vi "Teleop.vi"(10 "Match Info":T1={"Autonomous Elapsed Seconds"=0.0, "TeleOp Elapsed Seconds"=0.0, "Disabled Elapsed Seconds"=0.0, "Visited Autonomous"=FALSE, "Visited TeleOp"=FALSE, "Visited Disabled"=FALSE, "Autonomous Settings"={"Autonomous Style"=enum."Independent", "VI Refnum"=refnum}}, 11 "Call Context":T2) -> ()   [LabVIEW 2020]
doc: "This VI is called for each TeleOp packet received from the DS where the robot is not disabled. It is often used to read from the joysticks and update I/O or to update setpoints for timed control loops. It should complete and return within 20 milliseconds or it may miss DS packets."
uses:
  <vilib>/Rock Robotics/Network Tables/NT Read Boolean.vi
  <vilib>/Rock Robotics/Network Tables/NT Read Number.vi
  Robot Global Data.vi
  <vilib>/Rock Robotics/Network Tables/NT Write Numeric Array.vi
  <vilib>/Rock Robotics/WPI/ThirdParty/Phoenix-LabVIEW/Motor Controller/Controls/CTRE_Phoenix_MotorControl_ControlMode.ctl
  <vilib>/Rock Robotics/WPI/Solenoid/Deprecated/WPI_SolenoidSetBool.vi
  <vilib>/Rock Robotics/WPI/Solenoid/WPI_SolenoidValue.ctl
  <vilib>/Rock Robotics/Network Tables/NT Write Number.vi
  <vilib>/Rock Robotics/Network Tables/NT Write Boolean Array.vi
  <vilib>/Rock Robotics/WPI/Solenoid/WPI_SolenoidSetEnum.vi
  <vilib>/Rock Robotics/WPI/Solenoid/Deprecated/WPI_SolenoidGetBool.vi
  <vilib>/Rock Robotics/WPI/DriverStation/WPI_DriverStationMatch Info.ctl
  <vilib>/Rock Robotics/WPI/DriverStation/WPI_DriverStationDerivedRobotMode.ctl
panel:
  out "TargetValid 5":bool
  out "TargetValid 4":bool
  out "POVs":i16[](array[numeric])
  out "Sample Slider 0":dbl(slide) scale=0.0..5.0
  out "Sample Boolean 1":bool
  out "Sample Boolean 0":bool
  # "April tags"
  # "Retroreflective tape"
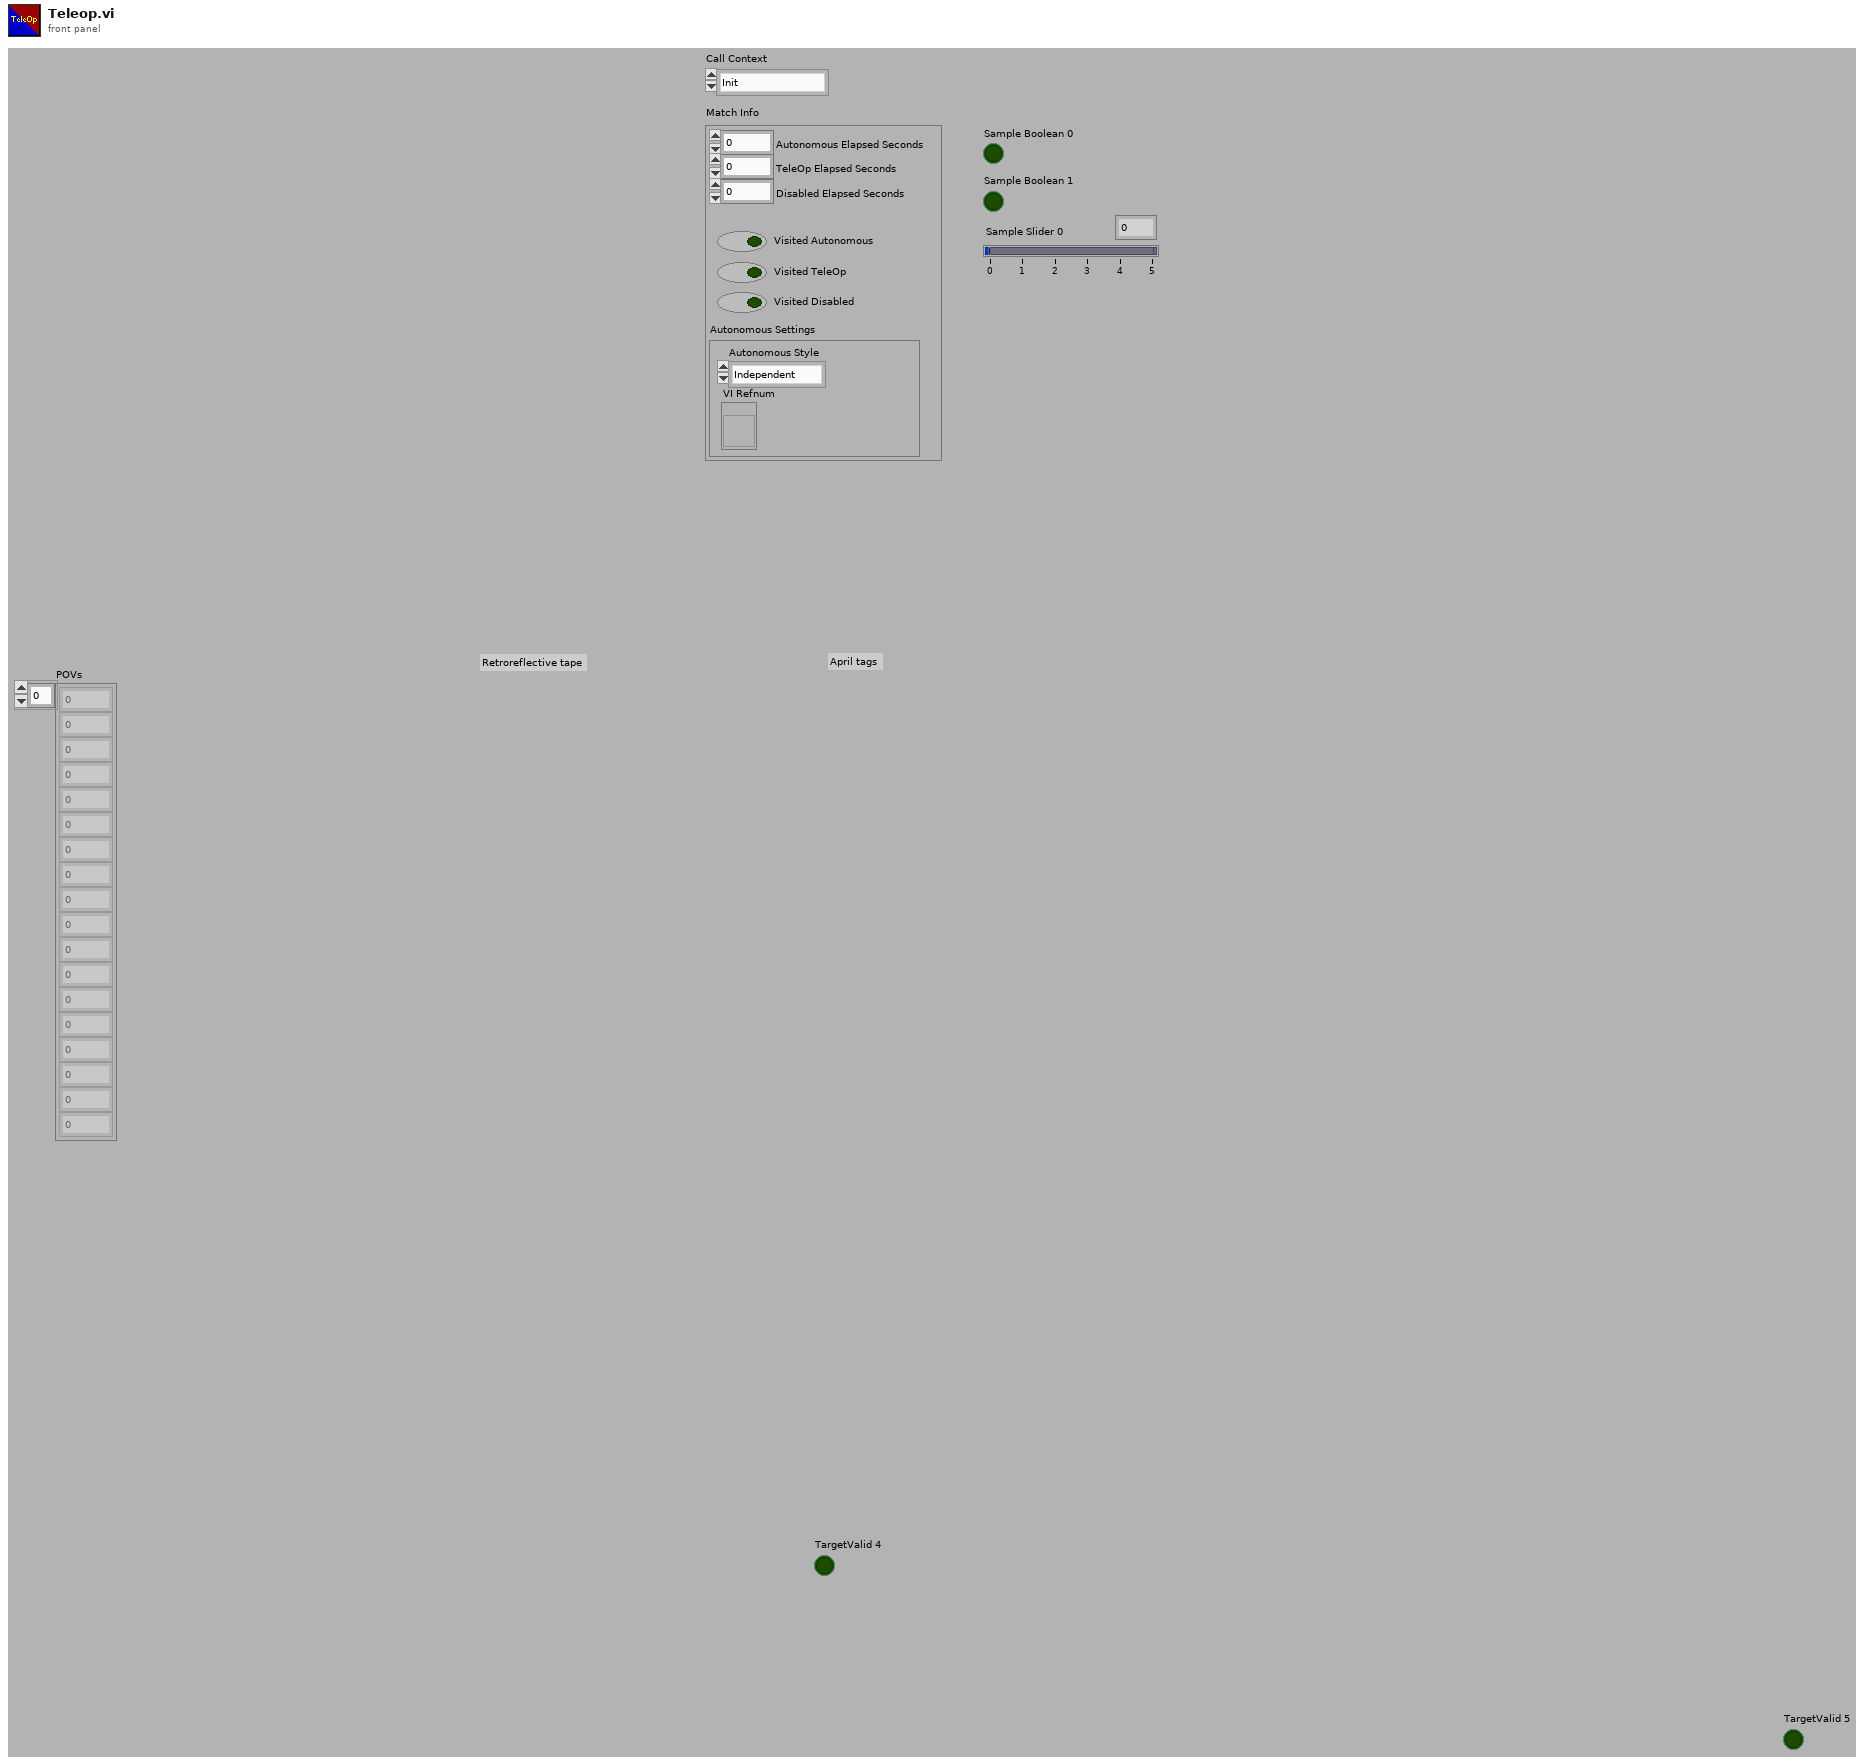
[diagram p1: front panel]
types:
  T1 = typedef "WPI_DriverStationMatch Info.ctl" = cluster{"Autonomous Elapsed Seconds":dbl, "TeleOp Elapsed Seconds":dbl, "Disabled Elapsed Seconds":dbl, "Visited Autonomous":bool, "Visited TeleOp":bool, "Visited Disabled":bool, "Autonomous Settings":cluster{"Autonomous Style":enum16{"Iterative", "Independent"}, "VI Refnum":refnum<vi>}}
  T2 = typedef "WPI_DriverStationDerivedRobotMode.ctl" = enum16{"Init", "Execute", "Stop"}
  T3 = typedef "WPI_SolenoidValue.ctl" = enum16{"Off", "On", "Forward", "Reverse"}
  T4 = cluster{"offsetAngle H":dbl, "offsetAngle V":dbl, "area":dbl, "skew":dbl}
  T5 = typedef "WPI_JoystickDevRef.ctl" = cluster{"Device":T6}
  T6 = typedef "WPI_JoystickDeviceEnum.ctl" = enum16{"USB 0", "USB 1", "USB 2", "USB 3", "USB 4", "USB 5"}
  T7 = cluster{"Buttons[0]":bool, "Buttons[1]":bool, "Buttons[2]":bool, "Buttons[3]":bool, "Buttons[4]":bool, "Buttons[5]":bool, "Buttons[6]":bool, "Buttons[7]":bool, "Buttons[8]":bool}
  T8 = cluster{"Axes[0]":dbl, "Axes[1]":dbl, "Axes[2]":dbl, "Axes[3]":dbl, "Axes[4]":dbl, "Axes[5]":dbl, "Axes[6]":dbl, "Axes[7]":dbl, "Axes[8]":dbl}
  T9 = typedef "WPI_RobotDriveDevRef.ctl" = cluster{"DevStatus":errorcluster, "Motors[]":T10[], "Square Inputs":bool, "Max Output":dbl}
  T10 = typedef "WPI_MotorControlDeviceRef.ctl" = cluster{"DeviceStatus":errorcluster, "Type":T11, "PWM":cluster{"PWM Channel":T12, "DeadBand":T13}, "CAN":cluster{"Device Number":u8, "SetOutput VI Ref":variant, "GetOutput VI Ref":variant, "Enable VI Ref":variant, "Disable VI Ref":variant, "Data":variant}, "Invert":bool, "DIO PWM":cluster{"PWM \"Enable\" Channel":T12, "DIOChannel":T14, "PWM Rate":dbl}}
  T11 = typedef "WPI_MotorControlType.ctl" = enum16{"PWM", "CAN", "DIO PWM"}
  T12 = typedef "FPGA_DIOPWMChannel.ctl" = enum8{"PWM 0", "PWM 1", "PWM 2", "PWM 3", "PWM 4", "PWM 5", "PWM 6", "PWM 7", "PWM 8", "PWM 9", "PWM MXP 0", "PWM MXP 1", "PWM MXP 2", "PWM MXP 3", "PWM MXP 4", "PWM MXP 5", "PWM MXP 6", "PWM MXP 7", "PWM MXP 8", "PWM MXP 9", "Invalid"}
  T13 = typedef "WPI_PWMDeadband.ctl" = cluster{"Name":string, "maxPositivePwm":i32, "minPositivePwm":i32, "centerPwm":i32, "maxNegativePwm":i32, "minNegativePwm":i32, "angularRange":u16}
  T14 = typedef "FPGA_DIOChannel.ctl" = enum8{"DIO 0", "DIO 1", "DIO 2", "DIO 3", "DIO 4", "DIO 5", "DIO 6", "DIO 7", "DIO 8", "DIO 9", "DIO MXP 0", "DIO MXP 1", "DIO MXP 2", "DIO MXP 3", "DIO MXP 4", "DIO MXP 5", "DIO MXP 6", "DIO MXP 7", "DIO MXP 8", "DIO MXP 9", "DIO MXP 10", "DIO MXP 11", "DIO MXP 12", "DIO MXP 13", "DIO MXP 14", "DIO MXP 15", "SPI Port CS1", "SPI Port CS2", "SPI Port CS3", "SPI Port MISO", "SPI Port MOSI", "Invalid"}
  T15 = typedef "WPI_SolenoidDevRef.ctl" = cluster{"DevStatus":errorcluster, "Pneumatics Control Module":u8, "Forward Solenoid Channel":T16, "Reverse Solenoid Channel":T16}
  T16 = typedef "WPI_SolenoidChannel.ctl" = enum8{"Solenoid 0", "Solenoid 1", "Solenoid 2", "Solenoid 3", "Solenoid 4", "Solenoid 5", "Solenoid 6", "Solenoid 7", "Solenoid 8", "Solenoid 9", "Solenoid 10", "Solenoid 11", "Solenoid 12", "Solenoid 13", "Solenoid 14", "Solenoid 15", "Invalid"}
  T17 = typedef "CTRE_Phoenix_MotorControl_ControlMode.ctl" = u16
  T18 = cluster{"Motors[][0]":T10, "Motors[][1]":T10, "Motors[][2]":T10, "Motors[][3]":T10, "Motors[][4]":T10, "Motors[][5]":T10, "Motors[][6]":T10, "Motors[][7]":T10, "Motors[][8]":T10}
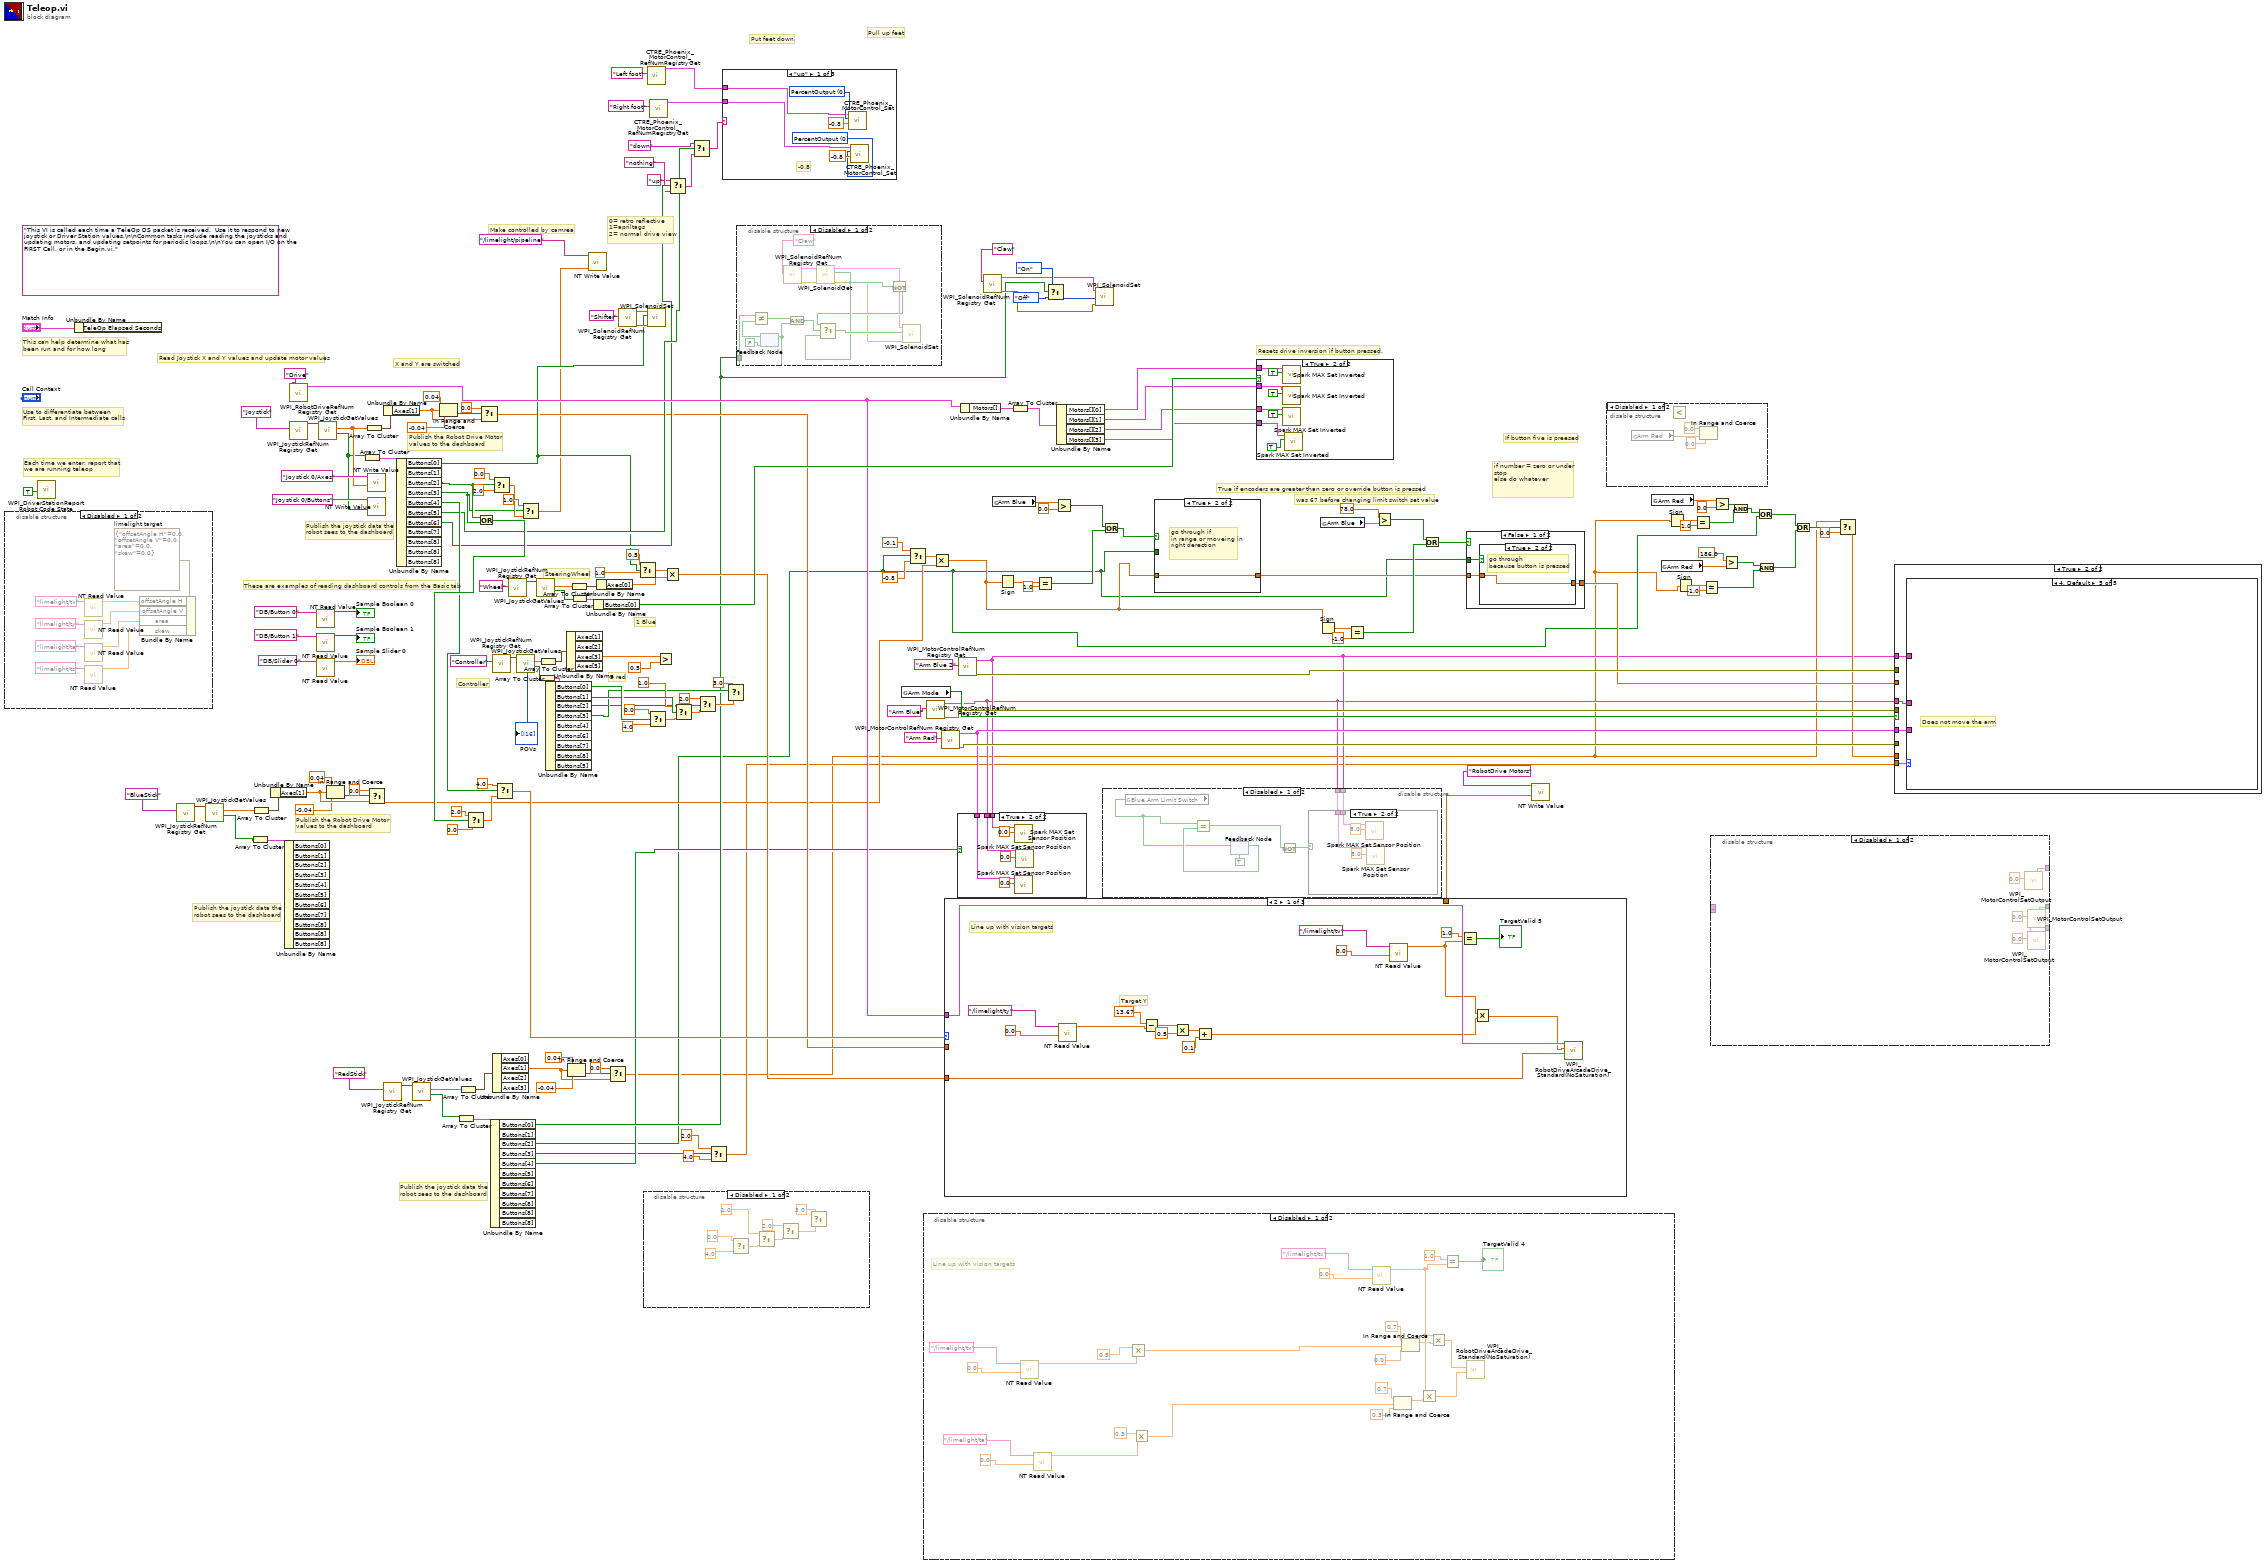
[diagram p0: block diagram]
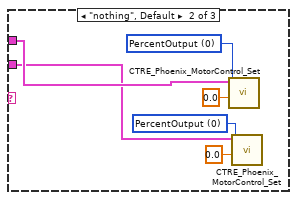
[diagram p8: hidden frame]
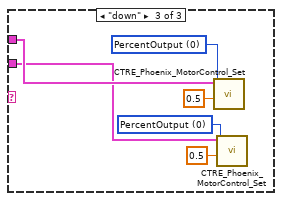
[diagram p9: hidden frame]
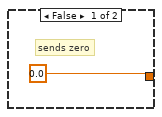
[diagram p10: hidden frame]
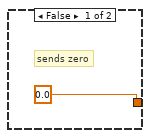
[diagram p13: hidden frame]
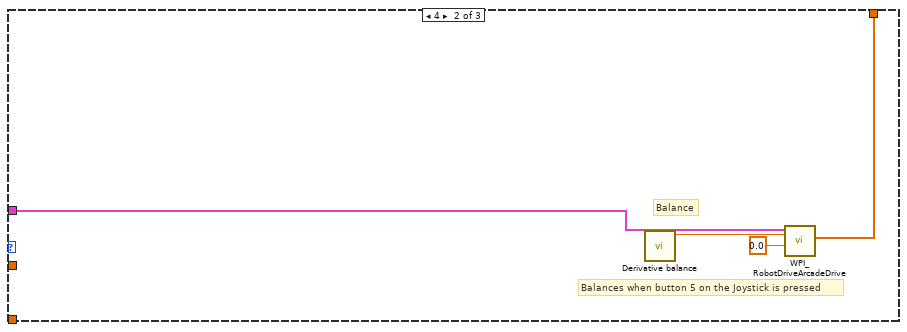
[diagram p17: hidden frame]
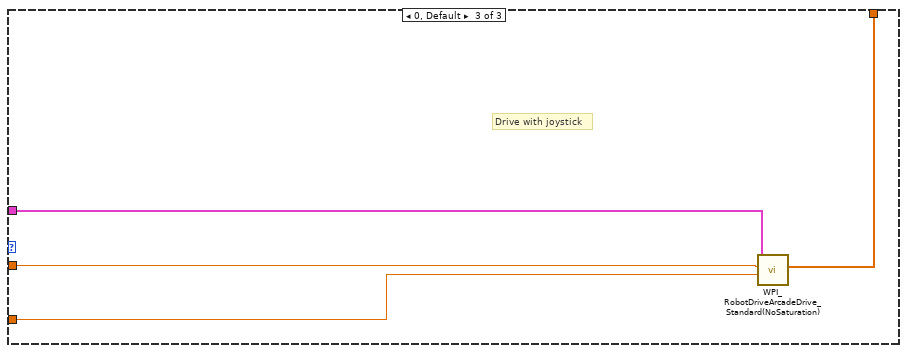
[diagram p18: hidden frame]
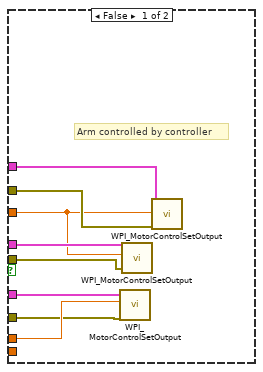
[diagram p19: hidden frame]
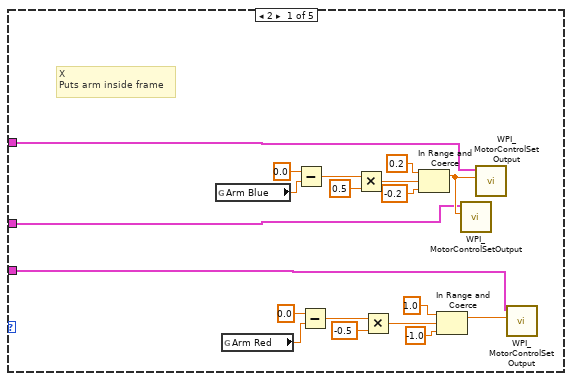
[diagram p20: hidden frame]
diagram:
  (unwired) "This VI is called each time a TeleOp DS packet is received.  Use it to respond to new joystick or Driver Station values.\n\nCommon tasks include reading the joysticks and updating motors, and updating setpoints for periodic loops.\n\nYou can open I/O on the FIRST Call, or in the Begin.vi."
  # "Publish the Robot Drive Motor\nvalues to the dashboard"
  # "Publish the joystick data the\nrobot sees to the dashboard"
  # "Publish the joystick data the\nrobot sees to the dashboard"
  # "5 red"
  # "1 Blue"
  # "X and Y are switched"
  # "Put feet down"
  # "Pull up feet"
  # "was 67 before changing limit switch set value"
  # "True if encoders are greater than zero or override button is pressed"
  # "if number = zero or under\nstop\nelse do whatever"
  # "If button five is preesed"
  # "Resets drive inversion if button pressed."
  # "0= retro reflective\n1=apriltags\n2= normal drive view"
  # "Make controlled by camrea"
  # "SteeringWheel"
  # "Controller"
  # "These are examples of reading dashboard controls from the Basic tab"
  # "Publish the Robot Drive Motor\nvalues to the dashboard"
  # "Publish the joystick data the\nrobot sees to the dashboard"
  # "Each time we enter, report that\nwe are running teleop"
  # "Use to differentiate between\nFirst, Last, and Intermediate calls"
  # "This can help determine what has\nbeen run and for how long"
  # "Read Joystick X and Y values and update motor values"
  n1 = disable-structure shown="Disabled" {
    frame Disabled {
      w185 = T4 {"offsetAngle H"=0.0, "offsetAngle V"=0.0, "area"=0.0, "skew"=0.0}  # limelight target
      n2 = call-poly <vilib>:"NT Read Value.vi"("name"="limelight/tx" ("Name")) -> ("value"=w184:dbl)  [unwired: 8 in, 2 out]
      n3 = call-poly <vilib>:"NT Read Value.vi"("name"="limelight/ty" ("Name")) -> ("value"=w183:dbl)  [unwired: 8 in, 2 out]
      n4 = call-poly <vilib>:"NT Read Value.vi"("name"="limelight/ta" ("Name")) -> ("value"=w182:dbl)  [unwired: 8 in, 2 out]
      n5 = call-poly <vilib>:"NT Read Value.vi"("name"="limelight/ts" ("Name")) -> ("value"=w181:dbl)  [unwired: 8 in, 2 out]
      n6 = Bundle By Name(cluster=w185, "offsetAngle H"=w184, "offsetAngle V"=w183, "area"=w182, "skew"=w181) -> ()  [unwired: 1 out]
    }
    frame Enabled {
    }
  }
  n7 = call <vilib>:"WPI_DriverStationReport Robot Code State.vi"("TeleOp"=TRUE ("Autonomous")) -> ()  [unwired: 10 in, 1 out]
  n8 = Unbundle By Name("Match Info") -> ()  [unwired: 1 out]
  n9 = call <vilib>:"WPI_JoystickRefNum Registry Get.vi"("refnum name"="BlueStick") -> ("JoystickDevRef"=w18:T5)  [unwired: 1 in, 9 out]
  n10 = call <vilib>:"WPI_JoystickGetValues.vi"("JoystickDevRef"=w18) -> ("Buttons"=w21:bool[], "Axes"=w19:dbl[])  [unwired: 6 in, 3 out]
  n11 = Array To Cluster(array=w21) -> (cluster=w22:T7)
  n12 = Array To Cluster(array=w19) -> (cluster=w20:T8)
  n13 = Unbundle By Name(w20) -> ("Axes[1]"=w26:dbl)
  n14 = Unbundle By Name(w22) -> ()  [unwired: 11 out]
  n15 = call <vilib>:"WPI_RobotDriveRefNum Registry Get.vi"("refnum name"="Drive") -> ("RobotDriveDevRef"=w108:T9)  [unwired: 1 in, 9 out]
  n16 = call <vilib>:"WPI_JoystickRefNum Registry Get.vi"("refnum name"="Joystick") -> ("JoystickDevRef"=w177:T5)  [unwired: 1 in, 9 out]
  n17 = call-poly <vilib>:"NT Read Value.vi"("name"="DB/Button 0" ("refnum name")) -> ("value"=→"Sample Boolean 0":bool)  [unwired: 8 in, 2 out]
  n18 = call-poly <vilib>:"NT Read Value.vi"("name"="DB/Slider 0" ("refnum name")) -> ("value"=→"Sample Slider 0":dbl)  [unwired: 8 in, 2 out]
  n19 = call-poly <vilib>:"NT Read Value.vi"("name"="DB/Button 1" ("refnum name")) -> ("value"=→"Sample Boolean 1":bool)  [unwired: 8 in, 2 out]
  n20 = call <vilib>:"WPI_JoystickGetValues.vi"("JoystickDevRef"=w177) -> ("Buttons"=w137:bool[], "Axes"=w166:dbl[])  [unwired: 6 in, 3 out]
  n21 = In Range and Coerce(upper limit=0.04, x=w26, lower limit=-0.04) -> (In Range?=w23:bool)  [unwired: 1 out]
  n22 = Array To Cluster(array=w137) -> (cluster=w136:T7)
  n23 = Array To Cluster(array=w166) -> (cluster=w165:T8)
  n24 = call-poly <vilib>:"NT Write Value.vi"("value"=w166, "name"="Joystick 0/Axes" ("Name")) -> ()  [unwired: 9 in, 1 out]
  n25 = call-poly <vilib>:"NT Write Value.vi"("value"=w137, "name"="Joystick 0/Buttons" ("Name")) -> ()  [unwired: 9 in, 1 out]
  n26 = Select(t=0.0, s=w23, f=w26) -> (s? t:f=w15:dbl)
  n27 = Unbundle By Name(w165) -> ("Axes[1]"=w39:dbl)
  n28 = call <vilib>:"WPI_JoystickRefNum Registry Get.vi"("refnum name"="RedStick") -> ("JoystickDevRef"=w31:T5)  [unwired: 1 in, 9 out]
  n29 = Unbundle By Name(w136) -> ("Buttons[0]"=w48:bool, "Buttons[2]"=w120:bool, "Buttons[3]"=w119:bool, "Buttons[4]"=w67:bool, "Buttons[5]"=w66:bool, "Buttons[6]"=w62:bool)  [unwired: 5 out]
  n30 = call <vilib>:"WPI_JoystickGetValues.vi"("JoystickDevRef"=w31) -> ("Buttons"=w28:bool[], "Axes"=w30:dbl[])  [unwired: 6 in, 3 out]
  n31 = In Range and Coerce(upper limit=0.04, x=w39, lower limit=-0.04) -> (In Range?=w43:bool)  [unwired: 1 out]
  n32 = Array To Cluster(array=w28) -> (cluster=w27:T7)
  n33 = Array To Cluster(array=w30) -> (cluster=w29:T8)
  n34 = Or(x=w120, y=w119) -> (x .or. y?=w118:bool)
  n35 = Select(t=2.0, s=w118, f=0.0) -> (s? t:f=w133:dbl)
  n36 = Select(t=0.0, s=w43, f=w39) -> (s? t:f=w38:dbl)
  n37 = Unbundle By Name(w27) -> ("Buttons[0]"=w16:bool, "Buttons[2]"=w13:bool, "Buttons[3]"=w10:bool, "Buttons[4]"=w14:bool)  [unwired: 7 out]
  n38 = Select(t=0.0, s=w120, f=2.0) -> (s? t:f=w121:dbl)
  n39 = call <vilib>:"WPI_JoystickRefNum Registry Get.vi"("refnum name"="Controller") -> ("JoystickDevRef"=w159:T5)  [unwired: 9 in, 1 out]
  n40 = Unbundle By Name(w29) -> ("Axes[1]"=w5:dbl)  [unwired: 3 out]
  n41 = Select(t=4.0, s=w67, f=w133) -> (s? t:f=w131:dbl)
  n42 = call <vilib>:"WPI_JoystickRefNum Registry Get.vi"("refnum name"="Wheel") -> ("JoystickDevRef"=w163:T5)  [unwired: 9 in, 1 out]
  n43 = call <vilib>:"WPI_JoystickGetValues.vi"("JoystickDevRef"=w159) -> ("Buttons"=w156:bool[], "Axes"=w158:dbl[], "POVs"=→"POVs":i16[])  [unwired: 6 in, 2 out]
  n44 = Select(t=1.0, s=w119, f=w121) -> (s? t:f=w33:dbl)
  n45 = call <vilib>:"WPI_JoystickGetValues.vi"("JoystickDevRef"=w163) -> ("Buttons"=w113:bool[], "Axes"=w162:dbl[])  [unwired: 6 in, 3 out]
  n46 = Array To Cluster(array=w156) -> (cluster=w155:T7)
  n47 = Array To Cluster(array=w158) -> (cluster=w157:T8)
  n48 = Unbundle By Name(w155) -> ("Buttons[0]"=w153:bool, "Buttons[1]"=w148:bool, "Buttons[2]"=w1:bool, "Buttons[3]"=w141:bool)  [unwired: 5 out]
  n49 = Unbundle By Name(w157) -> ("Axes[3]"=w125:dbl)  [unwired: 3 out]
  n50 = In Range and Coerce(upper limit=0.04, x=w5, lower limit=-0.04) -> (In Range?=w6:bool)  [unwired: 1 out]
  n51 = Array To Cluster(array=w162) -> (cluster=w161:T8)
  n52 = Array To Cluster(array=w113) -> (cluster=w112:T7)
  n53 = call-poly <vilib>:"NT Write Value.vi"("value"=w33, "name"="/limelight/pipeline" ("Name")) -> ()  [unwired: 9 in, 1 out]
  n54 = Unbundle By Name(w112) -> ("Buttons[0]"=w111:bool)
  n55 = Unbundle By Name(w161) -> ("Axes[0]"=w47:dbl)
  n56 = Select(t=0.0, s=w6, f=w5) -> (s? t:f=w4:dbl)
  n57 = call <vilib>:"WPI_SolenoidRefNum Registry Get.vi"("refnum name"="Shifter") -> ("error out"=w129:errorcluster, "SolenoidDevRef"=w128:T15)  [unwired: 9 in]
  n58 = Select(t=0.5, s=w48, f=1.0) -> (s? t:f=w49:dbl)
  n59 = disable-structure shown="Disabled" {
    frame Disabled {
      n60 = Select(t=0.0, f=4.0) -> (s=w201:bool, s? t:f=w198:dbl)
      n61 = Select(t=1.0, f=w198) -> (s=w196:bool, s? t:f=w197:dbl)
      n62 = Select(t=2.0, f=w197) -> (s? t:f=w191:dbl)  [unwired: 1 in]
      n63 = Select(t=3.0, f=w191) -> (s=w193:bool, s? t:f=w190:dbl)
    }
    frame Enabled {
    }
  }
  n64 = call <vilib>:"CTRE_Phoenix_MotorControl_RefNumRegistryGet.vi"("refnum name"="Left foot") -> ("PhoenixMotorControlDevRef"=w56:T10)  [unwired: 9 in, 1 out]
  n65 = call-poly <vilib>:"WPI_SolenoidSet.vi"("error in (no error)"=w129, "Value"=w48, "SolenoidDevRef"=w128) -> ()  [unwired: 7 in, 2 out]
  n66 = call <vilib>:"CTRE_Phoenix_MotorControl_RefNumRegistryGet.vi"("refnum name"="Right foot") -> ("PhoenixMotorControlDevRef"=w57:T10)  [unwired: 9 in, 1 out]
  n67 = Select(t=0.0, s=w153, f=4.0) -> (s? t:f=w150:dbl)
  n68 = Greater?(x=w125, y=0.5) -> ()  [unwired: 1 out]
  n69 = Multiply(x=w49, y=w47) -> (x*y=w46:dbl)
  n70 = Select(t="up", s=w62, f="nothing") -> (s? t:f=w63:string)
  n71 = Select(t=1.0, s=w148, f=w150) -> (s? t:f=w149:dbl)
  n72 = Select(t="down", s=w66, f=w63) -> (s? t:f=w64:string)
  n73 = Select(t=2.0, s=w1, f=w149) -> (s? t:f=w139:dbl)
  n74 = Select(t=2.0, s=w10, f=4.0) -> (s? t:f=w9:dbl)
  n75 = case shown="\"up\"" w64 {
    tunnel: w57 -> [w203 w208 w214]
    tunnel: w56 -> [w202 w209 w215]
    frame "up" {
      w206 = T17 0 items=["PercentOutput"=0, "Position"=1, "Velocity"=2, "Current"=3, "Follower"=5, "MotionProfile"=6, "MotionMagic"=7, "MotionProfileArc"=10, "Disabled"=15] ("Control Mode")
      w204 = T17 0 items=["PercentOutput"=0, "Position"=1, "Velocity"=2, "Current"=3, "Follower"=5, "MotionProfile"=6, "MotionMagic"=7, "MotionProfileArc"=10, "Disabled"=15] ("Control Mode")
      # "-0.8"
      n76 = call <vilib>:"CTRE_Phoenix_MotorControl_Set.vi"("Output"=-0.8, "Control Mode"=w204, "PhoenixMotorControlDevRef"=w202) -> ()  [unwired: 7 in, 2 out]
      n77 = call <vilib>:"CTRE_Phoenix_MotorControl_Set.vi"("Output"=-0.8, "Control Mode"=w206, "PhoenixMotorControlDevRef"=w203) -> ()  [unwired: 7 in, 2 out]
    }
    frame "nothing", Default {
      w211 = T17 0 items=["PercentOutput"=0, "Position"=1, "Velocity"=2, "Current"=3, "Follower"=5, "MotionProfile"=6, "MotionMagic"=7, "MotionProfileArc"=10, "Disabled"=15] ("Control Mode")
      w213 = T17 0 items=["PercentOutput"=0, "Position"=1, "Velocity"=2, "Current"=3, "Follower"=5, "MotionProfile"=6, "MotionMagic"=7, "MotionProfileArc"=10, "Disabled"=15] ("Control Mode")
      n78 = call <vilib>:"CTRE_Phoenix_MotorControl_Set.vi"("Output"=0.0, "Control Mode"=w213, "PhoenixMotorControlDevRef"=w209) -> ()  [unwired: 7 in, 2 out]
      n79 = call <vilib>:"CTRE_Phoenix_MotorControl_Set.vi"("Output"=0.0, "Control Mode"=w211, "PhoenixMotorControlDevRef"=w208) -> ()  [unwired: 7 in, 2 out]
    }
    frame "down" {
      w217 = T17 0 items=["PercentOutput"=0, "Position"=1, "Velocity"=2, "Current"=3, "Follower"=5, "MotionProfile"=6, "MotionMagic"=7, "MotionProfileArc"=10, "Disabled"=15] ("Control Mode")
      w219 = T17 0 items=["PercentOutput"=0, "Position"=1, "Velocity"=2, "Current"=3, "Follower"=5, "MotionProfile"=6, "MotionMagic"=7, "MotionProfileArc"=10, "Disabled"=15] ("Control Mode")
      n80 = call <vilib>:"CTRE_Phoenix_MotorControl_Set.vi"("Output"=0.5, "Control Mode"=w219, "PhoenixMotorControlDevRef"=w215) -> ()  [unwired: 7 in, 2 out]
      n81 = call <vilib>:"CTRE_Phoenix_MotorControl_Set.vi"("Output"=0.5, "Control Mode"=w217, "PhoenixMotorControlDevRef"=w214) -> ()  [unwired: 7 in, 2 out]
    }
  }
  n82 = Select(t=3.0, s=w141, f=w139) -> ()  [unwired: 1 out]
  n83 = disable-structure shown="Disabled" {
    disable-tunnel: w16 -> [w227 _]
    frame Disabled {
      n84 = feedback #1(FALSE ("x > y?")) -> (w231:bool)
      n85 = Not Equal?(x=w227, y=w231) -> (x != y?=w229:bool)
      n86 = feedback-in #1(w227) -> ()
      n87 = call <vilib>:"WPI_SolenoidRefNum Registry Get.vi"("refnum name"="Claw") -> ("error out"=w225:errorcluster, "SolenoidDevRef"=w226:T15)  [unwired: 9 in]
      n88 = And(x=w229, y=w227) -> (x .and. y?=w228:bool)
      n89 = call-poly <vilib>:"WPI_SolenoidGet.vi"("error in (no error)"=w225, "SolenoidDevRef"=w226) -> ("error out"=w220:errorcluster, "Value"=w223:bool, "SolenoidDevRef"=w221:T15)  [unwired: 7 in]
      n90 = Not(x=w223) -> (.not. x?=w222:bool)
      n91 = Select(t=w222, s=w228, f=w223) -> (s? t:f=w232:bool)
      n92 = call-poly <vilib>:"WPI_SolenoidSet.vi"("error in (no error)"=w220, "Value"=w232, "SolenoidDevRef"=w221) -> ()  [unwired: 7 in, 2 out]
    }
    frame Enabled {
    }
  }
  n93 = global read "Robot Global Data.vi" "Arm Mode"() -> (w154:bool)
  n94 = Select(t=-0.1, s=w13, f=-0.8) -> (s? t:f=w37:dbl)
  n95 = disable-structure shown="Disabled" {
    frame Disabled {
      # "Line up with vision targets"
      n96 = call-poly <vilib>:"NT Read Value.vi"("default value"=0.0 ("Default Value"), "name"="/limelight/tx" ("Name")) -> ("value"=w234:dbl)  [unwired: 7 in, 2 out]
      n97 = call-poly <vilib>:"NT Read Value.vi"("default value"=0.0 ("Default Value"), "name"="/limelight/ta" ("Name")) -> ("value"=w238:dbl)  [unwired: 7 in, 2 out]
      n98 = Multiply(x=0.5, y=w234) -> (x*y=w233:dbl)
      n99 = Multiply(x=0.3, y=w238) -> (x*y=w237:dbl)
      n100 = call-poly <vilib>:"NT Read Value.vi"("default value"=0.0 ("Default Value"), "name"="/limelight/tv" ("Name")) -> ("value"=w245:dbl)  [unwired: 7 in, 2 out]
      n101 = In Range and Coerce(upper limit=0.7, x=w237, lower limit=0.3) -> (coerced(x)=w244:dbl)  [unwired: 1 out]
      n102 = In Range and Coerce(upper limit=0.7, x=w233, lower limit=0.0) -> (coerced(x)=w243:dbl)  [unwired: 1 out]
      n103 = Multiply(x=w245, y=w244) -> (x*y=w247:dbl)
      n104 = Multiply(x=w245, y=w243) -> (x*y=w246:dbl)
      n105 = Equal?(x=1.0, y=w245) -> (x = y?=→"TargetValid 4":bool)
      n106 = call <vilib>:"WPI_RobotDriveArcadeDrive_Standard(NoSaturation).vi"("Y axis value"=w247, "X axis value"=w246) -> ()  [unwired: 2 in, 8 out]
    }
    frame Enabled {
    }
  }
  n107 = call <vilib>:"WPI_MotorControlRefNum Registry Get.vi"("refnum name"="Arm Blue") -> ("error out"=w144:errorcluster, "MotorControlDevRef"=w68:T10)  [unwired: 9 in]
  n108 = Multiply(x=w37, y=w15) -> (x*y=w34:dbl)
  n109 = call <vilib>:"WPI_MotorControlRefNum Registry Get.vi"("refnum name"="Arm Red") -> ("error out"=w142:errorcluster, "MotorControlDevRef"=w114:T10)  [unwired: 9 in]
  n110 = case shown="2" w131 {
    tunnel: w108 -> [w270 w276 w280]
    tunnel: w38 -> [_ _ w279]
    tunnel: w46 -> [w256 _ w278]
    tunnel: [_ w275 w277] -> w130
    frame 2 {
      # "Target Y"
      # "Line up with vision targets"
      n111 = call-poly <vilib>:"NT Read Value.vi"("default value"=0.0 ("Default Value"), "name"="/limelight/ty" ("Name")) -> ("value"=w260:dbl)  [unwired: 7 in, 2 out]
      n112 = Subtract(x=13.67, y=w260) -> (x-y=w269:dbl)
      n113 = Multiply(x=w269, y=0.5) -> (x*y=w261:dbl)
      n114 = Add(x=w261, y=0.1) -> (x+y=w257:dbl)
      n115 = call-poly <vilib>:"NT Read Value.vi"("default value"=0.0 ("Default Value"), "name"="/limelight/tv" ("Name")) -> ("value"=w264:dbl)  [unwired: 7 in, 2 out]
      n116 = Equal?(x=1.0, y=w264) -> (x = y?=→"TargetValid 5":bool)
      n117 = Multiply(x=w264, y=w257) -> (x*y=w263:dbl)
      n118 = call <vilib>:"WPI_RobotDriveArcadeDrive_Standard(NoSaturation).vi"("Y axis value"=w256, "X axis value"=w263, "RobotDriveDevRef"=w270) -> ()  [unwired: 1 in, 8 out]
    }
    frame 4 {
      # "Balances when button 5 on the Joystick is pressed"
      # "Balance"
      n119 = call "Derivative balance.vi"() -> ("Motor Power"=w274:dbl)  [unwired: 11 in]
      n120 = call-poly <vilib>:"WPI_RobotDriveArcadeDrive.vi"("Y axis value"=0.0, "X axis value"=w274, "RobotDriveDevRef"=w276) -> ("Motor Values"=w275:dbl[])  [unwired: 6 in, 2 out]
    }
    frame 0, Default {
      # "Drive with joystick"
      n121 = call <vilib>:"WPI_RobotDriveArcadeDrive_Standard(NoSaturation).vi"("Y axis value"=w278, "X axis value"=w279, "RobotDriveDevRef"=w280) -> ("Motor Values"=w277:dbl[])  [unwired: 1 in, 7 out]
    }
  }
  n122 = call <vilib>:"WPI_MotorControlRefNum Registry Get.vi"("refnum name"="Arm Blue 2") -> ("error out"=w115:errorcluster, "MotorControlDevRef"=w69:T10)  [unwired: 9 in]
  n123 = case shown="True" w14 {
    tunnel: w69 -> [_ w286]
    tunnel: w68 -> [_ w285]
    tunnel: w114 -> [_ w284]
    frame False {
    }
    frame True {
      n124 = call <vilib>:"Spark MAX Set Sensor Position.vi"("Position"=0.0, "MotorControlDeviceRef"=w286) -> ()  [unwired: 8 in, 2 out]
      n125 = call <vilib>:"Spark MAX Set Sensor Position.vi"("Position"=0.0, "MotorControlDeviceRef"=w284) -> ()  [unwired: 8 in, 2 out]
      n126 = call <vilib>:"Spark MAX Set Sensor Position.vi"("Position"=0.0, "MotorControlDeviceRef"=w285) -> ()  [unwired: 8 in, 2 out]
    }
  }
  n127 = Unbundle By Name(w108) -> ("Motors[]"=w110:T10[])
  n128 = call <vilib>:"WPI_SolenoidRefNum Registry Get.vi"("refnum name"="Claw") -> ("error out"=w50:errorcluster, "SolenoidDevRef"=w51:T15)  [unwired: 9 in]
  n129 = global read "Robot Global Data.vi" "Arm Blue"() -> (w103:dbl)
  n130 = Sign(1:w34) -> (0:w100:dbl)
  n131 = Array To Cluster(array=w110) -> (cluster=w109:T18)
  n132 = Equal?(x=w100, y=1.0) -> (x = y?=w98:bool)
  n133 = Select(t=WPI_SolenoidValue."On" ("Value"), s=w16, f=WPI_SolenoidValue."Off" ("Value")) -> (s? t:f=w54:T3)
  n134 = Greater?(x=w103, y=0.0) -> (0:w102:bool)
  n135 = Unbundle By Name(w109) -> ("Motors[][0]"=w107:T10, "Motors[][1]"=w105:T10, "Motors[][2]"=w104:T10, "Motors[][3]"=w106:T10)
  n136 = call-poly <vilib>:"WPI_SolenoidSet.vi"("error in (no error)"=w50, "Value"=w54, "SolenoidDevRef"=w51) -> ()  [unwired: 7 in, 2 out]
  n137 = Or(x=w102, y=w98) -> (x .or. y?=w97:bool)
  n138 = disable-structure shown="Disabled" {
    disable-tunnel: w69 -> [w292 _]
    disable-tunnel: w68 -> [w291 _]
    frame Disabled {
      n139 = global read "Robot Global Data.vi" "Blue Arm Limit Switch"() -> (w288:bool)
      n140 = feedback #2(TRUE) -> (w289:bool)
      n141 = Equal?(x=w288, y=w289) -> (x = y?=w287:bool)
      n142 = feedback-in #2(w288) -> ()
      n143 = Not(x=w287) -> (.not. x?=w293:bool)
      n144 = case shown="True" w293 {
        tunnel: w292 -> [_ w297]
        tunnel: w291 -> [_ w296]
        frame False {
        }
        frame True {
          n145 = call <vilib>:"Spark MAX Set Sensor Position.vi"("Position"=8.0, "MotorControlDeviceRef"=w297) -> ()  [unwired: 8 in, 2 out]
          n146 = call <vilib>:"Spark MAX Set Sensor Position.vi"("Position"=8.0, "MotorControlDeviceRef"=w296) -> ()  [unwired: 8 in, 2 out]
        }
      }
    }
    frame Enabled {
    }
  }
  n147 = case shown="True" w97 {
    tunnel: w13 -> [w300 _]
    tunnel: [w299 w303] -> w89
    tunnel: w34 -> [w298 w303]
    frame False {
      n148 = case shown="True" w300 {
        tunnel: [0.0 w302] -> w299
        tunnel: w298 -> [_ w302]
        frame False {
          # "sends zero"
        }
        frame True {
          # "go through\nbecause button is pressed"
        }
      }
    }
    frame True {
      # "go through if\nin range or moveing in right derection"
    }
  }
  n149 = case shown="True" w111 {
    tunnel: w107 -> [_ w311]
    tunnel: w106 -> [_ w306]
    tunnel: w105 -> [_ w305]
    tunnel: w104 -> [_ w304]
    frame False {
    }
    frame True {
      n150 = call <vilib>:"Spark MAX Set Inverted.vi"("Inverted (F)"=TRUE, "MotorControlDeviceRef in"=w311) -> ()  [unwired: 8 in, 2 out]
      n151 = call <vilib>:"Spark MAX Set Inverted.vi"("Inverted (F)"=TRUE, "MotorControlDeviceRef in"=w305) -> ()  [unwired: 8 in, 2 out]
      n152 = call <vilib>:"Spark MAX Set Inverted.vi"("Inverted (F)"=TRUE, "MotorControlDeviceRef in"=w304) -> ()  [unwired: 8 in, 2 out]
      n153 = call <vilib>:"Spark MAX Set Inverted.vi"("Inverted (F)"=TRUE, "MotorControlDeviceRef in"=w306) -> ()  [unwired: 8 in, 2 out]
    }
  }
  n154 = Sign(1:w34) -> (0:w95:dbl)
  n155 = global read "Robot Global Data.vi" "Arm Blue"() -> (w91:dbl)
  n156 = Equal?(x=w95, y=-1.0) -> (x = y?=w93:bool)
  n157 = Greater?(x=78.0 ("y"), y=w91) -> (0:w96:bool)
  n158 = Or(x=w96, y=w93) -> (x .or. y?=w92:bool)
  n159 = case shown="False" w92 {
    tunnel: w13 -> [w314 _]
    tunnel: [w313 w317] -> w88
    tunnel: w89 -> [w312 w317]
    frame False {
      n160 = case shown="True" w314 {
        tunnel: [0.0 w316] -> w313
        tunnel: w312 -> [_ w316]
        frame False {
          # "sends zero"
        }
        frame True {
          # "go through\nbecause button is pressed"
        }
      }
    }
    frame True {
      # "go through if\nin range or moveing in right derection"
    }
  }
  n161 = call-poly <vilib>:"NT Write Value.vi"("value"=w130, "name"="RobotDrive Motors" ("Name")) -> ()  [unwired: 9 in, 1 out]
  n162 = disable-structure shown="Disabled" {
    frame Disabled {
      n163 = global read "Robot Global Data.vi" "Arm Red"() -> (w318:dbl)
      n164 = Less?() -> ()  [unwired: 2 in, 1 out]
      n165 = In Range and Coerce(upper limit=0.0, x=w318, lower limit=0.0) -> ()  [unwired: 2 out]
    }
    frame Enabled {
    }
  }
  n166 = global read "Robot Global Data.vi" "Arm Red"() -> (w87:dbl)
  n167 = global read "Robot Global Data.vi" "Arm Red"() -> (w81:dbl)
  n168 = Sign(1:w4) -> (0:w85:dbl)
  n169 = Sign(1:w4) -> (0:w83:dbl)
  n170 = Equal?(x=w85, y=1.0) -> (x = y?=w78:bool)
  n171 = Equal?(x=w83, y=-1.0) -> (x = y?=w77:bool)
  n172 = disable-structure shown="Disabled" {
    disable-tunnel: [w324 _] -> _
    disable-tunnel: _ -> [w324 _]
    disable-tunnel: _ -> [w323 _]
    disable-tunnel: _ -> [w322 _]
    disable-tunnel: _ -> [w321 _]
    frame Disabled {
      n173 = call <vilib>:"WPI_MotorControlSetOutput.vi"("Output"=0.0, "MotorControlDevRef"=w321) -> ()  [unwired: 7 in, 3 out]
      n174 = call <vilib>:"WPI_MotorControlSetOutput.vi"("Output"=0.0, "MotorControlDevRef"=w323) -> ()  [unwired: 7 in, 3 out]
      n175 = call <vilib>:"WPI_MotorControlSetOutput.vi"("Output"=0.0, "MotorControlDevRef"=w322) -> ()  [unwired: 7 in, 3 out]
    }
    frame Enabled {
    }
  }
  n176 = Greater?(x=w87, y=0.0) -> (0:w79:bool)
  n177 = Greater?(x=186.0 ("y"), y=w81) -> (0:w76:bool)
  n178 = And(x=w79, y=w78) -> (x .and. y?=w75:bool)
  n179 = Or(x=w75, y=w13) -> (x .or. y?=w73:bool)
  n180 = And(x=w76, y=w77) -> (x .and. y?=w74:bool)
  n181 = Or(x=w73, y=w74) -> (x .or. y?=w72:bool)
  n182 = Select(t=w4, s=w72, f=0.0) -> (s? t:f=w70:dbl)
  n183 = case shown="True" w154 {
    tunnel: w70 -> [w335 _]
    tunnel: w144 -> [w334 _]
    tunnel: w68 -> [w333 w336]
    tunnel: w142 -> [w332 _]
    tunnel: w114 -> [w331 w338]
    tunnel: w9 -> [_ w339]
    tunnel: w69 -> [w330 w337]
    tunnel: w115 -> [w329 _]
    tunnel: w88 -> [w328 _]
    frame False {
      # "Arm controlled by controller"
      n184 = call <vilib>:"WPI_MotorControlSetOutput.vi"("error in (no error)"=w332, "Output"=w335, "MotorControlDevRef"=w331) -> ()  [unwired: 6 in, 3 out]
      n185 = call <vilib>:"WPI_MotorControlSetOutput.vi"("error in (no error)"=w334, "Output"=w328, "MotorControlDevRef"=w333) -> ()  [unwired: 6 in, 3 out]
      n186 = call <vilib>:"WPI_MotorControlSetOutput.vi"("error in (no error)"=w329, "Output"=w328, "MotorControlDevRef"=w330) -> ()  [unwired: 6 in, 3 out]
    }
    frame True {
      n187 = case shown="4, Default" w339 {
        tunnel: w338 -> [w340 w359 w378 w399 _]
        tunnel: w337 -> [w342 w361 w380 w398 _]
        tunnel: w336 -> [w341 w360 w379 w397 _]
        frame 2 {
          # "X\nPuts arm inside frame"
          n188 = global read "Robot Global Data.vi" "Arm Blue"() -> (w356:dbl)
          n189 = global read "Robot Global Data.vi" "Arm Red"() -> (w351:dbl)
          n190 = Subtract(x=0.0, y=w356) -> (x-y=w357:dbl)
          n191 = Subtract(x=0.0, y=w351) -> (x-y=w358:dbl)
          n192 = Multiply(x=w357, y=0.5) -> (x*y=w352:dbl)
          n193 = Multiply(x=w358, y=-0.5) -> (x*y=w353:dbl)
          n194 = In Range and Coerce(upper limit=0.2, x=w352, lower limit=-0.2) -> (coerced(x)=w355:dbl)  [unwired: 1 out]
          n195 = In Range and Coerce(upper limit=1.0, x=w353, lower limit=-1.0) -> (coerced(x)=w354:dbl)  [unwired: 1 out]
          n196 = call <vilib>:"WPI_MotorControlSetOutput.vi"("Output"=w355, "MotorControlDevRef"=w341) -> ()  [unwired: 7 in, 3 out]
          n197 = call <vilib>:"WPI_MotorControlSetOutput.vi"("Output"=w355, "MotorControlDevRef"=w342) -> ()  [unwired: 7 in, 3 out]
          n198 = call <vilib>:"WPI_MotorControlSetOutput.vi"("Output"=w354, "MotorControlDevRef"=w340) -> ()  [unwired: 7 in, 3 out]
        }
        frame 3 {
          # "Y\nPlaces piece on top row"
          n199 = global read "Robot Global Data.vi" "Arm Blue"() -> (w375:dbl)
          n200 = global read "Robot Global Data.vi" "Arm Red"() -> (w370:dbl)
          n201 = Subtract(x=67.2, y=w375) -> (x-y=w376:dbl)
          n202 = Subtract(x=145.592, y=w370) -> (x-y=w377:dbl)
          n203 = Multiply(x=w376, y=0.5) -> (x*y=w371:dbl)
          n204 = Multiply(x=w377, y=-0.5) -> (x*y=w372:dbl)
          n205 = In Range and Coerce(upper limit=0.2, x=w371, lower limit=-0.2) -> (coerced(x)=w374:dbl)  [unwired: 1 out]
          n206 = In Range and Coerce(upper limit=1.0, x=w372, lower limit=-1.0) -> (coerced(x)=w373:dbl)  [unwired: 1 out]
          n207 = call <vilib>:"WPI_MotorControlSetOutput.vi"("Output"=w374, "MotorControlDevRef"=w360) -> ()  [unwired: 7 in, 3 out]
          n208 = call <vilib>:"WPI_MotorControlSetOutput.vi"("Output"=w374, "MotorControlDevRef"=w361) -> ()  [unwired: 7 in, 3 out]
          n209 = call <vilib>:"WPI_MotorControlSetOutput.vi"("Output"=w373, "MotorControlDevRef"=w359) -> ()  [unwired: 7 in, 3 out]
        }
        frame 1 {
          # "B\nPlaces piece on middle row"
          n210 = global read "Robot Global Data.vi" "Arm Blue"() -> (w394:dbl)
          n211 = global read "Robot Global Data.vi" "Arm Red"() -> (w389:dbl)
          n212 = Subtract(x=19.238, y=w394) -> (x-y=w395:dbl)
          n213 = Subtract(x=135.831, y=w389) -> (x-y=w396:dbl)
          n214 = Multiply(x=w395, y=0.5) -> (x*y=w390:dbl)
          n215 = Multiply(x=w396, y=-0.5) -> (x*y=w391:dbl)
          n216 = In Range and Coerce(upper limit=0.2, x=w390, lower limit=-0.2) -> (coerced(x)=w393:dbl)  [unwired: 1 out]
          n217 = In Range and Coerce(upper limit=1.0, x=w391, lower limit=-1.0) -> (coerced(x)=w392:dbl)  [unwired: 1 out]
          n218 = call <vilib>:"WPI_MotorControlSetOutput.vi"("Output"=w393, "MotorControlDevRef"=w379) -> ()  [unwired: 7 in, 3 out]
          n219 = call <vilib>:"WPI_MotorControlSetOutput.vi"("Output"=w393, "MotorControlDevRef"=w380) -> ()  [unwired: 7 in, 3 out]
          n220 = call <vilib>:"WPI_MotorControlSetOutput.vi"("Output"=w392, "MotorControlDevRef"=w378) -> ()  [unwired: 7 in, 3 out]
        }
        frame 0 {
          # "A\nPlaces piece on bottom row"
          n221 = global read "Robot Global Data.vi" "Arm Blue"() -> (w413:dbl)
          n222 = global read "Robot Global Data.vi" "Arm Red"() -> (w408:dbl)
          n223 = Subtract(x=33.3568, y=w413) -> (x-y=w414:dbl)
          n224 = Subtract(x=34.7616, y=w408) -> (x-y=w415:dbl)
          n225 = Multiply(x=w414, y=0.5) -> (x*y=w409:dbl)
          n226 = Multiply(x=w415, y=-0.5) -> (x*y=w410:dbl)
          n227 = In Range and Coerce(upper limit=0.2, x=w409, lower limit=-0.2) -> (coerced(x)=w412:dbl)  [unwired: 1 out]
          n228 = In Range and Coerce(upper limit=1.0, x=w410, lower limit=-1.0) -> (coerced(x)=w411:dbl)  [unwired: 1 out]
          n229 = call <vilib>:"WPI_MotorControlSetOutput.vi"("Output"=w412, "MotorControlDevRef"=w397) -> ()  [unwired: 7 in, 3 out]
          n230 = call <vilib>:"WPI_MotorControlSetOutput.vi"("Output"=w412, "MotorControlDevRef"=w398) -> ()  [unwired: 7 in, 3 out]
          n231 = call <vilib>:"WPI_MotorControlSetOutput.vi"("Output"=w411, "MotorControlDevRef"=w399) -> ()  [unwired: 7 in, 3 out]
        }
        frame 4, Default {
          # "Does not move the arm"
        }
      }
    }
  }
